vi "gearCalculator.vi"(0 "VISA Refnum in":refnum<visa-resource-name>, 11 "error in (no error)":errorcluster) -> (4 "steps/button Array":dbl[][](array[numeric]), 6 "No Keys":bool, 8 "KeyCodeName":string[](array[string]), 10 "cycle":dbl, 15 "error out":errorcluster)   [LabVIEW 2018]
uses:
  Global_usbComm.vi
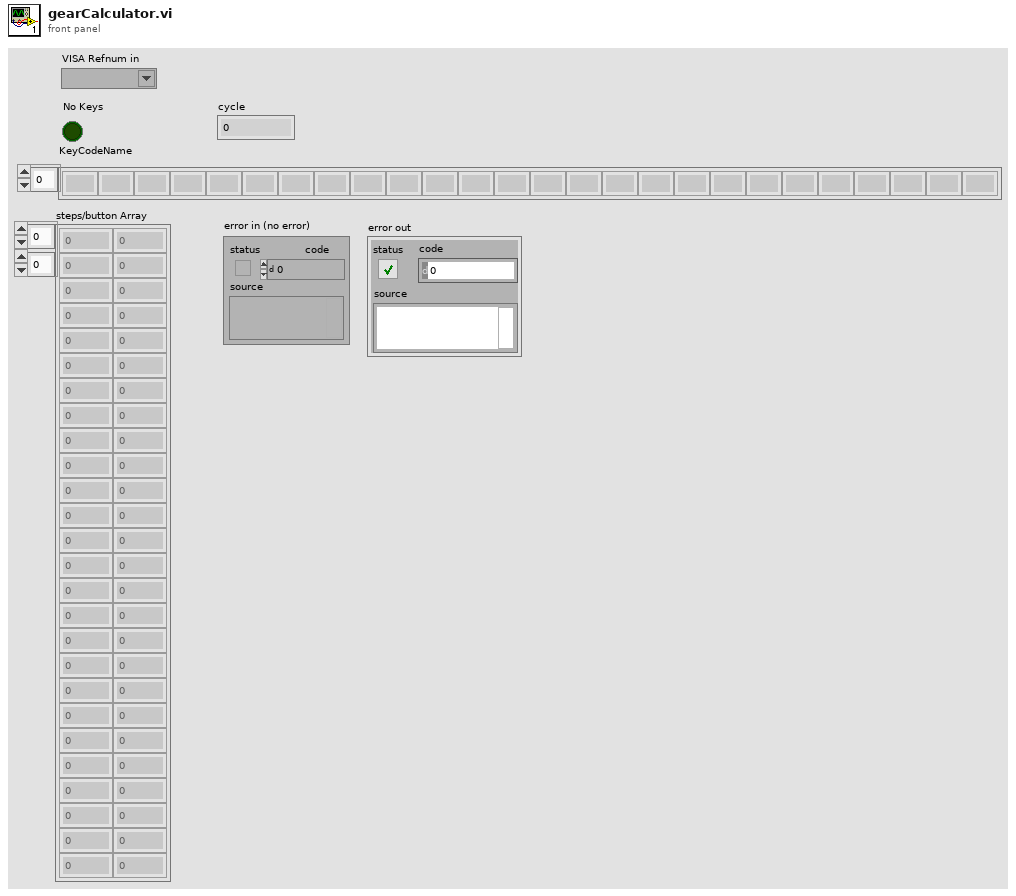
[diagram p1: front panel]
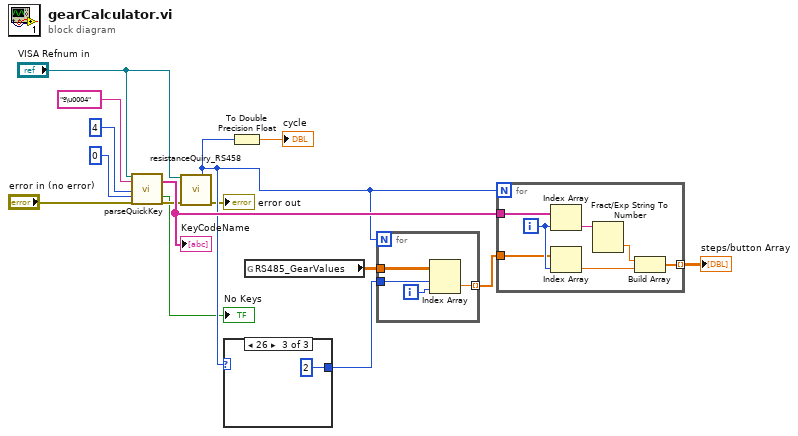
[diagram p0: block diagram]
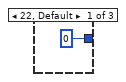
[diagram p2: hidden frame]
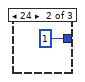
[diagram p3: hidden frame]
diagram:
  n1 = call "parseQuickKey.vi"("VISA resource name"="VISA Refnum in", "write buffer"="º\u0004", "y"=4, "x"=0 ("y"), "error in (no error)"="error in (no error)") -> ("KeyCodeName"=w14:string[], "No Keys"=→"No Keys":bool, "error out"=w6:errorcluster)  [unwired: 10 in, 2 out]
  "KeyCodeName" <- w14
  n2 = call "resistanceQuiry_RS458.vi"("VISA resource name"="VISA Refnum in", "error in (no error)"=w6) -> ("resistMax"=w8:u32, "error out"=→"error out":errorcluster)  [unwired: 7 in, 5 out]
  n3 = case shown="26" w8 {
    tunnel: [0 1 2] -> w9
    frame 22, Default {
    }
    frame 24 {
    }
    frame 26 {
    }
  }
  n4 = To Double Precision Float(number=w8) -> (double precision float=→"cycle":dbl)
  n5 = global read "Global_usbComm.vi" "RS485_GearValues"() -> (w2:dbl[][])
  n6 = for {
    N: w8 -> [_]
    tunnel: w2 -> [w22]
    tunnel: w9 -> [w20]
    tunnel: [w19] -> w7 mode=indexing
    i -> [w21]
    n7 = Index Array(array=w22, index (row)=w20, index (col)=w21) -> (element=w19:dbl)
  }
  n8 = for {
    N: w8 -> [_]
    tunnel: [w29] -> w15 mode=indexing
    tunnel: w14 -> [w28]
    tunnel: w7 -> [w24]
    i -> [w25]
    n9 = Index Array(array=w28, index=w25) -> (element=w27:string)
    n10 = Index Array(array=w24, index=w25) -> (element=w23:dbl)
    n11 = Fract/Exp String To Number(string=w27) -> (number=w26:dbl)  [unwired: 3 in, 1 out]
    n12 = Build Array(w26, w23) -> (w29:dbl[])
  }
  "steps/button Array" <- w15
